vi "TEMOCR-Initialize Hardware.vi"(5 "Params":T2, 11 "error in (no error)":errorcluster) -> (8 "AO":T1, 15 "error out":errorcluster)   [LabVIEW 2015]
uses:
  Typedefs/TEMOCR-Parameters.ctl
  Typedefs/TEMOCR-Probe.ctl
  Typedefs/TEMOCR-Elicitor.ctl
  Human Studies/SFM Frontend/LV Source/Typedefs/HSTS-Transducer.ctl
  Typedefs/TEMOCR-Sequence.ctl
  Typedefs/TEMOCR-Analysis.ctl
  Typedefs/TEMOCR-AO Data.ctl
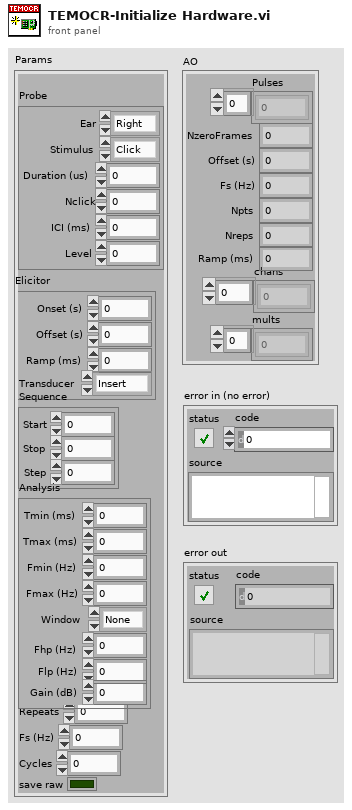
[diagram p1: front panel]
types:
  T1 = typedef "TEMOCR-AO Data.ctl" = cluster{"Pulses":dbl[], "Fs (Hz)":dbl, "Npts":i32, "mults":dbl[], "chans":i32[], "Nreps":i32, "NzeroFrames":i32, "Offset (s)":dbl, "Ramp (ms)":dbl}
  T2 = typedef "TEMOCR-Parameters.ctl" = cluster{"Probe":T3, "Elicitor":T4, "Sequence":T6, "Analysis":T7, "Repeats":i32, "Fs (Hz)":dbl, "Cycles":i32, "save raw":bool}
  T3 = typedef "TEMOCR-Probe.ctl" = cluster{"Ear":enum16{"Right", "Left"}, "Stimulus":enum16{"Click", "Chirp"}, "Duration (us)":dbl, "Nclick":i32, "ICI (ms)":dbl, "Level":dbl}
  T4 = typedef "TEMOCR-Elicitor.ctl" = cluster{"Onset (s)":dbl, "Offset (s)":dbl, "Ramp (ms)":dbl, "Transducer":T5}
  T5 = typedef "HSTS-Transducer.ctl" = enum16{"Insert", "TDH-39", "HD300", "ER-10X"}
  T6 = typedef "TEMOCR-Sequence.ctl" = cluster{"Start":dbl, "Stop":dbl, "Step":dbl}
  T7 = typedef "TEMOCR-Analysis.ctl" = cluster{"Tmin (ms)":dbl, "Tmax (ms)":dbl, "Fmin (Hz)":dbl, "Fmax (Hz)":dbl, "Window":enum16{"None", "Hanning", "Hamming"}, "Fhp (Hz)":dbl, "Flp (Hz)":dbl, "Gain (dB)":dbl}
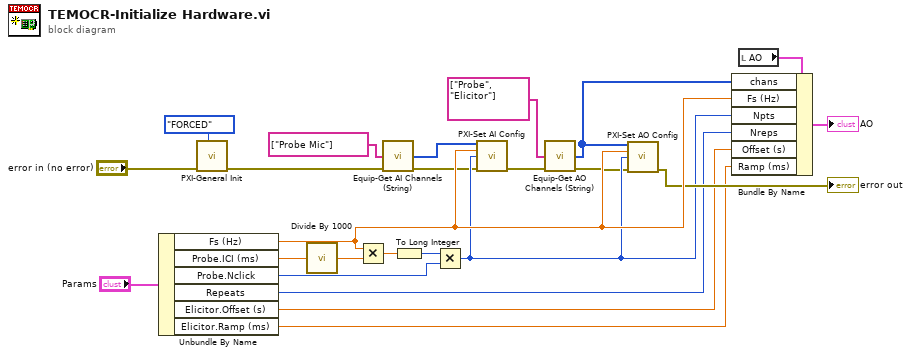
[diagram p0: block diagram]
diagram:
  n1 = Unbundle By Name("Params") -> ("Fs (Hz)"=w18:dbl, "Probe.ICI (ms)"=w22:dbl, "Probe.Nclick"=w11:i32, "Repeats"=w14:i32, "Elicitor.Offset (s)"=w10:dbl, "Elicitor.Ramp (ms)"=w9:dbl)
  n2 = call "PXI-General Init.vi"("Double Buffer Mode"=enum32{"OFF", "ENABLED", "FORCED"}."FORCED", "error in (no error)"="error in (no error)") -> ("error out"=w7:errorcluster)  [unwired: 9 in]
  n3 = call "Divide By 1000.vi"("X"=w22) -> ("X/1000"=w13:dbl)
  n4 = Multiply(x=w18, y=w13) -> (x*y=w21:dbl)
  n5 = call "Equip-Get AI Channels (String).vi"("Inputs"=string[] ["Probe Mic"], "error in (no error)"=w7) -> ("AI Channels"=w5:i32[], "error out"=w6:errorcluster)  [unwired: 12 in]
  n6 = To Long Integer(number=w21) -> (32bit integer=w17:i32)
  n7 = Multiply(x=w17, y=w11) -> (x*y=w12:i32)
  n8 = call "PXI-Set AI Config.vi"("AI Channels"=w5, "Sampling Rate (Hz)"=w18, "Buffer Size"=w12, "error in (no error)"=w6) -> ("error out"=w3:errorcluster)  [unwired: 11 in]
  n9 = call "Equip-Get AO Channels (String).vi"("Channel Names"=string[] ["Probe", "Elicitor"], "error in (no error)"=w3) -> ("AO Channels"=w1:i32[], "error out"=w2:errorcluster)  [unwired: 12 in]
  n10 = call "PXI-Set AO Config.vi"("AO Channels"=w1, "Sampling Rate (Hz)"=w18, "Buffer Size"=w12, "error in (no error)"=w2) -> ("error out"=→"error out":errorcluster)  [unwired: 11 in]
  n11 = local read "AO"() -> (w19:T1)
  n12 = Bundle By Name(cluster=w19, "chans"=w1, "Fs (Hz)"=w18, "Npts"=w12, "Nreps"=w14, "Offset (s)"=w10, "Ramp (ms)"=w9) -> (→"AO":T1)
